vi "WriteAmplifierUncalibratedOffset.vi"(8 "error in (no error)":errorcluster, 10 "Uncalibrated Offset":dbl, 11 "AmplifierSim in":refnum<class "AmplifierSim.lvclass">) -> (0 "error out":errorcluster, 3 "AmplifierSim out":refnum<class "AmplifierSim.lvclass">)   [LabVIEW 2017, in "AmplifierSim.lvclass"]
uses:
  AmplifierSim.lvclass
  AmplifierSim.lvclass/AmplifierSim.ctl
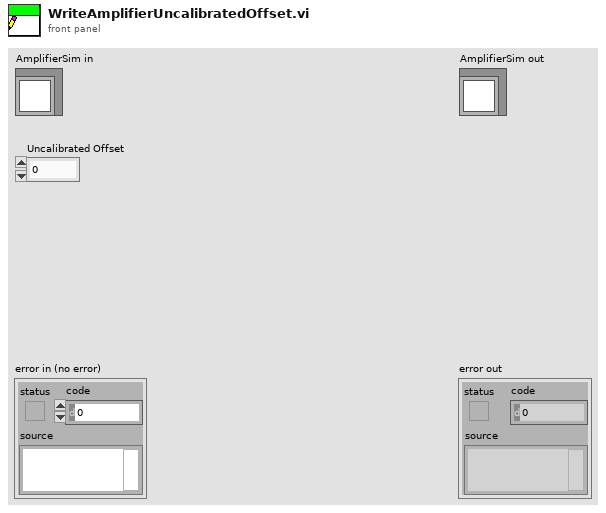
[diagram p1: front panel]
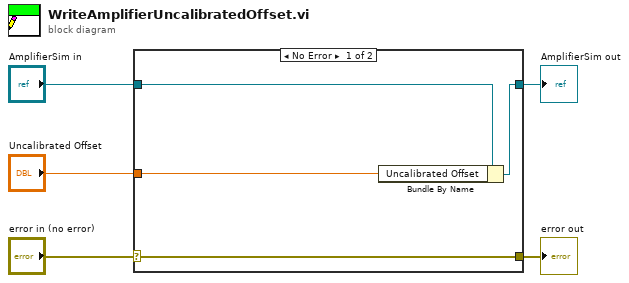
[diagram p0: block diagram]
diagram:
  n1 = case shown="No Error" "error in (no error)" {
    selector: "error in (no error)" -> [w9 w10]
    tunnel: [w9 w10] -> w4
    tunnel: [w7 w11] -> w2
    tunnel: "AmplifierSim in" -> [w8 w11]
    tunnel: "Uncalibrated Offset" -> [w6 _]
    frame No Error {
      n2 = Bundle By Name(cluster=w8, "Uncalibrated Offset"=w6) -> (w7:refnum<class "AmplifierSim.lvclass">)
    }
    frame Error {
    }
  }
  "error out" <- w4
  "AmplifierSim out" <- w2
